vi "Untitled 1 (SubVI).vi"(9 "Texture 3":T1 {"v" min=0 max=1 step=0.1; "u" min=0 max=1 step=0.1}, 10 "Texture 2":T1 {"v" min=0 max=1 step=0.1; "u" min=0 max=1 step=0.1}, 11 "Texture 1":T1 {"v" min=0 max=1 step=0.1; "u" min=0 max=1 step=0.1}) -> (0 "Height Delta":sgl, 1 "y start":sgl, 2 "Width Delta":sgl, 3 "x start":sgl)   [LabVIEW 2022 SP3]
uses:
  UV.ctl
  Raster.lvlib
panel:
  in  "Height Delta 2":sgl
  out "Texel Start Col (u)":sgl
  out "Texels In Widest Row (u)":sgl
  in  "u Delta":sgl
  out "Texels In Highest Col (v)":sgl
  out "Texel Start Row (v)":sgl
  in  "v start":sgl
  in  "Texture Number Of Cols":i32
  in  "Texture Number Of Rows":i32
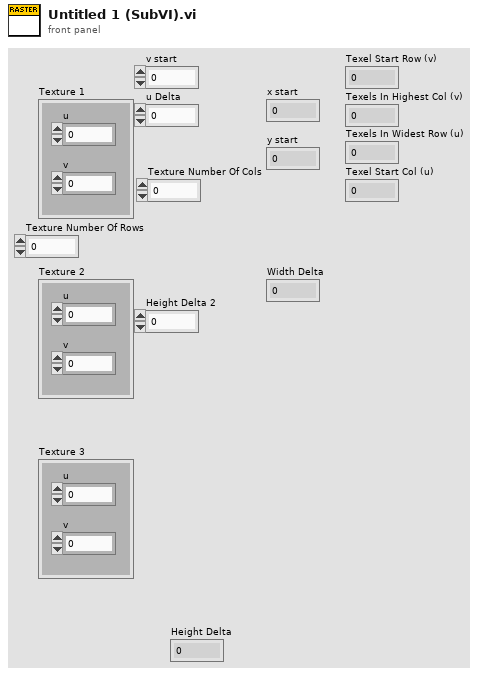
[diagram p1: front panel]
types:
  T1 = typedef "Raster.lvlib/UV.ctl" = cluster{"u":sgl, "v":sgl}
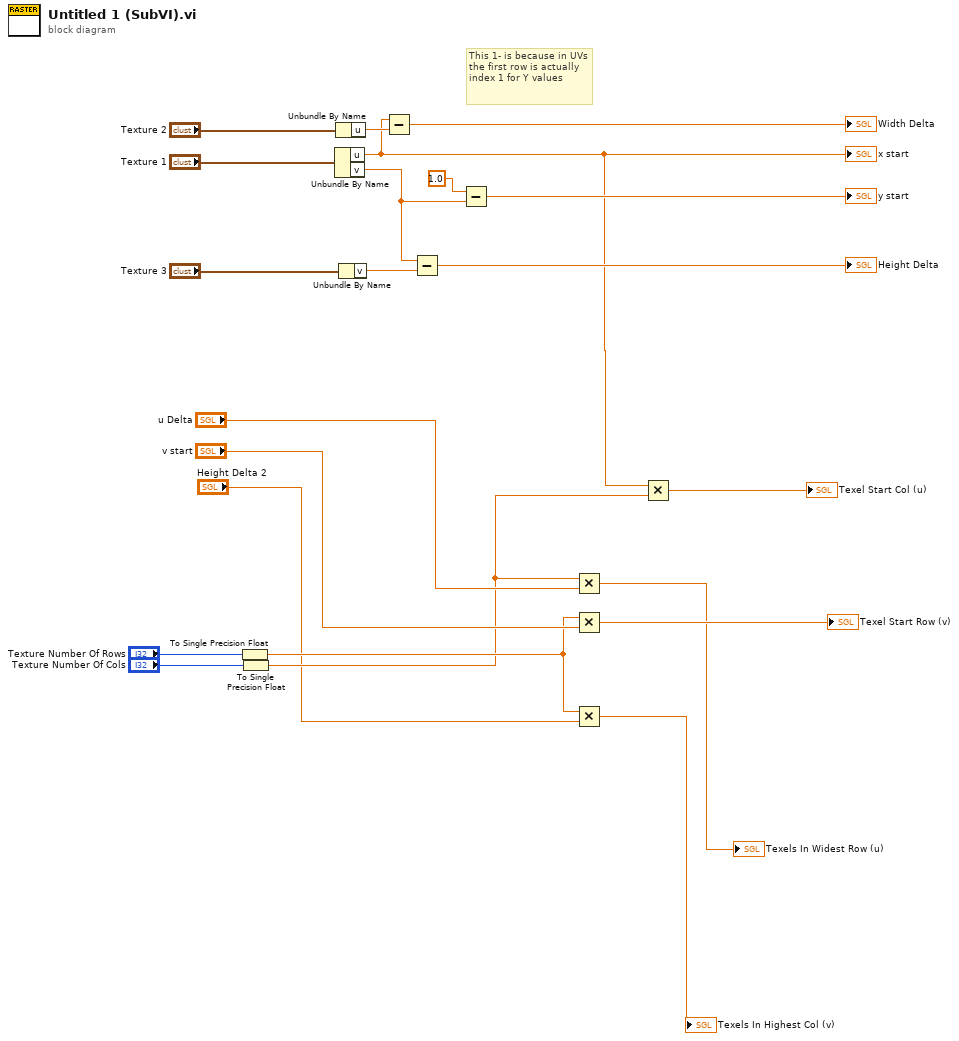
[diagram p0: block diagram]
diagram:
  # "This 1- is because in UVs the first row is actually index 1 for Y values"
  n1 = To Single Precision Float(number="Texture Number Of Rows") -> (single precision float=w8:sgl)
  n2 = To Single Precision Float(number="Texture Number Of Cols") -> (single precision float=w4:sgl)
  n3 = Unbundle By Name("Texture 1") -> ("u"=w1:sgl, "v"=w17:sgl)
  "x start" <- w1
  n4 = Unbundle By Name("Texture 2") -> ("u"=w21:sgl)
  n5 = Unbundle By Name("Texture 3") -> ("v"=w18:sgl)
  n6 = Subtract(x=w1, y=w21) -> (x-y=→"Width Delta":sgl)
  n7 = Subtract(x=w17, y=w18) -> (x-y=→"Height Delta":sgl)
  n8 = Subtract(x=sgl 1.0, y=w17) -> (x-y=→"y start":sgl)
  n9 = Multiply(x=w4, y="u Delta") -> (x*y=→"Texels In Widest Row (u)":sgl)
  n10 = Multiply(x=w8, y="v start") -> (x*y=→"Texel Start Row (v)":sgl)
  n11 = Multiply(x=w8, y="Height Delta 2") -> (x*y=→"Texels In Highest Col (v)":sgl)
  n12 = Multiply(x=w1, y=w4) -> (x*y=→"Texel Start Col (u)":sgl)
